vi "ampPdiv_Auto_subvi.vi"(9 "Amplitude/div":i32, 10 "Auto":bool, 11 "WaveformChart in":refnum<vi>) -> ()   [LabVIEW 2020]
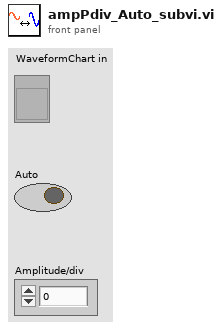
[diagram p1: front panel]
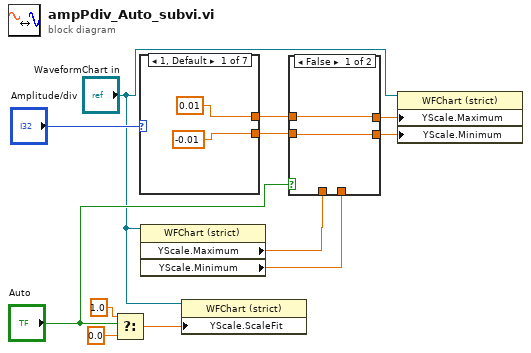
[diagram p0: block diagram]
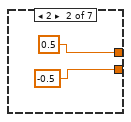
[diagram p3: hidden frame]
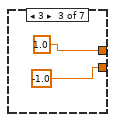
[diagram p4: hidden frame]
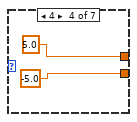
[diagram p5: hidden frame]
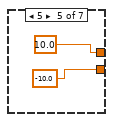
[diagram p6: hidden frame]
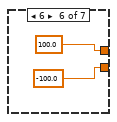
[diagram p7: hidden frame]
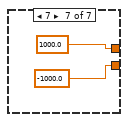
[diagram p8: hidden frame]
diagram:
  n1 = Select(t=1.0, s="Auto", f=0.0) -> (s? t:f=w5:dbl)
  n2 = case shown="1, Default" "Amplitude/div" {
    tunnel: [0.01 ("Y Scale.Range:Maximum") 0.5 ("Y Scale.Range:Maximum") 1.0 ("Y Scale.Range:Maximum") 5.0 ("Y Scale.Range:Maximum") 10.0 ("Y Scale.Range:Maximum") 100.0 ("Y Scale.Range:Maximum") 1000.0 ("Y Scale.Range:Maximum")] -> w8
    tunnel: [-0.01 ("Y Scale.Range:Minimum") -0.5 ("Y Scale.Range:Minimum") -1.0 ("Y Scale.Range:Minimum") -5.0 ("Y Scale.Range:Minimum") -10.0 ("Y Scale.Range:Minimum") -100.0 ("Y Scale.Range:Minimum") -1000.0 ("Y Scale.Range:Minimum")] -> w7
    frame 1, Default {
    }
    frame 2 {
    }
    frame 3 {
    }
    frame 4 {
    }
    frame 5 {
    }
    frame 6 {
    }
    frame 7 {
    }
  }
  n3 = property on="Property Node" class="WFChart (strict)"(reference="WaveformChart in") -> ("YScale.Maximum"=w9:dbl, "YScale.Minimum"=w10:dbl)  [unwired: 1 in, 2 out]
  n4 = property on="Property Node" class="WFChart (strict)"(reference="WaveformChart in", "YScale.ScaleFit"=w5) -> ()  [unwired: 1 in, 2 out]
  n5 = case shown="False" "Auto" {
    tunnel: w7 -> [w27 _]
    tunnel: w8 -> [w28 _]
    tunnel: w9 -> [_ w30]
    tunnel: w10 -> [_ w29]
    tunnel: [w28 w30] -> w11
    tunnel: [w27 w29] -> w12
    frame False {
    }
    frame True {
    }
  }
  n6 = property on="Property Node" class="WFChart (strict)"(reference="WaveformChart in", "YScale.Maximum"=w11, "YScale.Minimum"=w12) -> ()  [unwired: 1 in, 2 out]
